vi "Initialize RT.vi"(11 "Device Reference":T9 format="%.0x") -> (0 "error out":errorcluster, 3 "RT Data":T1 {"Compiled Data"."9759 RevB"."Settings"."ControlCals"."ThetaLH (deg)" format="%.3f"; "Compiled Data"."9759 RevB"."Settings"."ControlCals"."ULHLag (sec)" format="%.3f"; "Compiled Data"."9759 RevB"."Settings"."ControlCals"."USLag (sec)" format="%.3f"; "Compiled Data"."9759 RevB"."Settings"."ControlCals"."TLead (sec)" format="%.3f"; "Compiled Data"."9759 RevB"."Settings"."ControlCals"."TLag (sec)" format="%.3f"})   [LabVIEW 2015, in "NI 9759 RevB Custom Device.lvlib"]
uses:
  NI 9759 RevB Custom Device.lvlib
  <vilib>/NI Veristand/Custom Device API/Custom Device Item Ref.ctl
  Shared/Types/RT Data.ctl
  Shared/Types/Compiled Data.ctl
  Shared/Types/RT Init Data.ctl
  Shared/Types/RT Status.ctl
  Shared/Types/9759 RevB.ctl
  Shared/Types/FPGA Refs.ctl
  Shared/Types/Generic FPGA Ref.ctl
  Shared/Types/9759 RevB FPGA Ref.ctl
  Shared/9759 Properties.vi
  <vilib>/NI Veristand/Custom Device Tools/Custom Device Utility Library/Custom Device Utility Library.lvlib
  <vilib>/NI VeriStand/Custom Device API/Custom Device API.lvlib
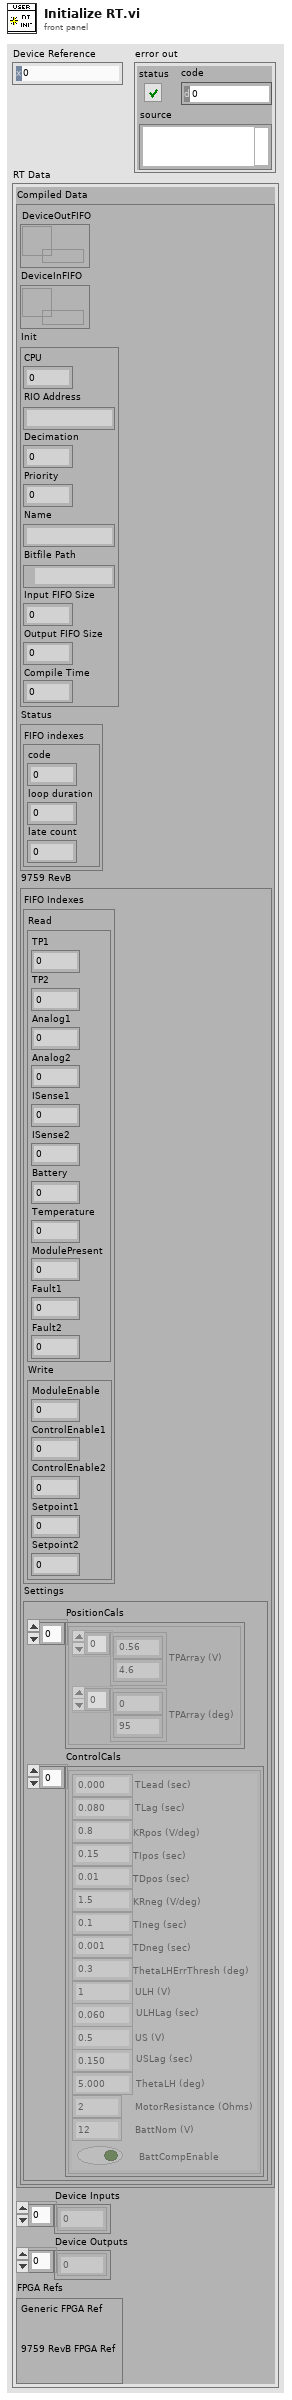
[diagram p1: front panel]
types:
  T1 = typedef "NI 9759 RevB Custom Device.lvlib/RT Data.ctl" = cluster{"Compiled Data":T2, "Device Inputs":dbl[], "Device Outputs":dbl[], "FPGA Refs":T6}
  T2 = typedef "NI 9759 RevB Custom Device.lvlib/Compiled Data.ctl" = cluster{"DeviceOutFIFO":refnum<k33>, "DeviceInFIFO":refnum<k33>, "Init":T3, "Status":T4, "9759 RevB":T5}
  T3 = typedef "NI 9759 RevB Custom Device.lvlib/RT Init Data.ctl" = cluster{"CPU":i32, "RIO Address":string, "Decimation":i32, "Priority":i32, "Name":string, "Bitfile Path":path, "Input FIFO Size":i32, "Output FIFO Size":i32, "Compile Time":dbl}
  T4 = typedef "NI 9759 RevB Custom Device.lvlib/RT Status.ctl" = cluster{"FIFO indexes":cluster{"code":i32, "loop duration":i32, "late count":i32}}
  T5 = typedef "NI 9759 RevB Custom Device.lvlib/9759 RevB.ctl" = cluster{"FIFO Indexes":cluster{"Read":cluster{"TP1":i32, "TP2":i32, "Analog1":i32, "Analog2":i32, "ISense1":i32, "ISense2":i32, "Battery":i32, "Temperature":i32, "ModulePresent":i32, "Fault1":i32, "Fault2":i32}, "Write":cluster{"ModuleEnable":i32, "ControlEnable1":i32, "ControlEnable2":i32, "Setpoint1":i32, "Setpoint2":i32}}, "Settings":cluster{"PositionCals":cluster{"TPArray (V)":sgl[], "TPArray (deg)":sgl[]}[], "ControlCals":cluster{"TLead (sec)":sgl, "TLag (sec)":sgl, "KRpos (V/deg)":sgl, "TIpos (sec)":sgl, "TDpos (sec)":sgl, "KRneg (V/deg)":sgl, "TIneg (sec)":sgl, "TDneg (sec)":sgl, "ThetaLHErrThresh (deg)":sgl, "ULH (V)":sgl, "ULHLag (sec)":sgl, "US (V)":sgl, "USLag (sec)":sgl, "ThetaLH (deg)":sgl, "MotorResistance (Ohms)":sgl, "BattNom (V)":sgl, "BattCompEnable":bool}[]}}
  T6 = typedef "NI 9759 RevB Custom Device.lvlib/FPGA Refs.ctl" = cluster{"Generic FPGA Ref":T7, "9759 RevB FPGA Ref":T8}
  T7 = typedef "NI 9759 RevB Custom Device.lvlib/Generic FPGA Ref.ctl" = refnum<k20>
  T8 = typedef "NI 9759 RevB Custom Device.lvlib/9759 RevB FPGA Ref.ctl" = refnum<k20>
  T9 = typedef "Custom Device API.lvlib/Custom Device Item Ref.ctl" = u64
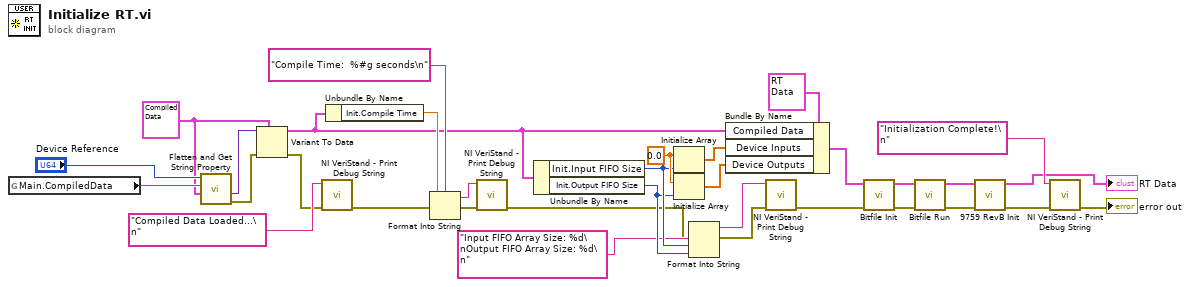
[diagram p0: block diagram]
diagram:
  w4 = T2 {"DeviceOutFIFO"=refnum, "DeviceInFIFO"=refnum, "Init"={"CPU"=0, "RIO Address"="", "Decimation"=0, "Priority"=0, "Name"="", "Bitfile Path"=path "", "Input FIFO Size"=0, "Output FIFO Size"=0, "Compile Time"=0.0}, "Status"={"FIFO indexes"={"code"=0, "loop duration"=0, "late count"=0}}, "9759 RevB"={"FIFO Indexes"={"Read"={"TP1"=0, "TP2"=0, "Analog1"=0, "Analog2"=0, "ISense1"=0, "ISense2"=0, "Battery"=0, "Temperature"=0, "ModulePresent"=0, "Fault1"=0, "Fault2"=0}, "Write"={"ModuleEnable"=0, "ControlEnable1"=0, "ControlEnable2"=0, "Setpoint1"=0, "Setpoint2"=0}}, "Settings"={"PositionCals"=[], "ControlCals"=[]}}} ("Compiled Data")
  w31 = 0.0 ("element")
  n1 = global read "9759 Properties.vi" "Main.CompiledData"() -> (w17:string)
  n2 = call "Flatten and Get String Property.vi"("Default Value"=w4, "Property Name"=w17, "Section Ref in"="Device Reference") -> ("error out"=w15:errorcluster, "Value"=w16:variant)  [unwired: 6 in, 1 out]
  n3 = Variant To Data(error in=w15, type=w4, Variant=w16) -> (data=w7:T2, error out=w14:errorcluster)
  n4 = call <vilib>:"NI VeriStand - Print Debug String.vi"("error in (no error)"=w14, "Message"="Compiled Data Loaded...\n") -> ("error out"=w12:errorcluster)  [unwired: 9 in]
  n5 = Unbundle By Name(w7) -> ("Init.Compile Time"=w11:dbl)
  n6 = Format Into String(format string="Compile Time:  %#g seconds\n" ("Message"), error in=w12, w11) -> (resulting string=w9:string, error out=w8:errorcluster)  [unwired: 1 in]
  n7 = call <vilib>:"NI VeriStand - Print Debug String.vi"("error in (no error)"=w8, "Message"=w9) -> ("error out"=w13:errorcluster)  [unwired: 9 in]
  n8 = Unbundle By Name(w7) -> ("Init.Input FIFO Size"=w23:i32, "Init.Output FIFO Size"=w22:i32)
  n9 = Initialize Array(w31, w23) -> (w33:dbl[])
  n10 = Initialize Array(w31, w22) -> (w32:dbl[])
  n11 = Format Into String(format string="Input FIFO Array Size: %d\nOutput FIFO Array Size: %d\n" ("initial string"), error in=w13, w23, w22) -> (resulting string=w24:string, error out=w20:errorcluster)  [unwired: 1 in]
  n12 = Bundle By Name(cluster=T1 {"Compiled Data"={"DeviceOutFIFO"=refnum, "DeviceInFIFO"=refnum, "Init"={"CPU"=0, "RIO Address"="", "Decimation"=0, "Priority"=0, "Name"="", "Bitfile Path"=path "", "Input FIFO Size"=0, "Output FIFO Size"=0, "Compile Time"=0.0}, "Status"={"FIFO indexes"={"code"=0, "loop duration"=0, "late count"=0}}, "9759 RevB"={"FIFO Indexes"={"Read"={"TP1"=0, "TP2"=0, "Analog1"=0, "Analog2"=0, "ISense1"=0, "ISense2"=0, "Battery"=0, "Temperature"=0, "ModulePresent"=0, "Fault1"=0, "Fault2"=0}, "Write"={"ModuleEnable"=0, "ControlEnable1"=0, "ControlEnable2"=0, "Setpoint1"=0, "Setpoint2"=0}}, "Settings"={"PositionCals"=[], "ControlCals"=[]}}}, "Device Inputs"=[], "Device Outputs"=[], "FPGA Refs"={"Generic FPGA Ref"=refnum, "9759 RevB FPGA Ref"=refnum}}, "Compiled Data"=w7, "Device Inputs"=w33, "Device Outputs"=w32) -> (w30:T1)
  n13 = call <vilib>:"NI VeriStand - Print Debug String.vi"("error in (no error)"=w20, "Message"=w24) -> ("error out"=w19:errorcluster)  [unwired: 9 in]
  n14 = call "Bitfile Init.vi"("error in"=w19, "RT Data In"=w30) -> ("error out"=w27:errorcluster, "RT Data Out"=w28:T1)  [unwired: 8 in]
  n15 = call "Bitfile Run.vi"("error in"=w27, "RT Data In"=w28) -> ("error out"=w2:errorcluster, "RT Data Out"=w5:T1)  [unwired: 8 in]
  n16 = call "9759 RevB Init.vi"("error in"=w2, "RT Data In"=w5) -> ("error out"=w1:errorcluster, "RT Data Out"=→"RT Data":T1)  [unwired: 8 in]
  n17 = call <vilib>:"NI VeriStand - Print Debug String.vi"("error in (no error)"=w1, "Message"="Initialization Complete!\n") -> ("error out"=→"error out":errorcluster)  [unwired: 9 in]
